vi "Write Error to File.vi"(8 "error in":errorcluster) -> ()   [LabVIEW 2021]
uses:
  <vilib>/Utility/xml.llb/Write to XML File(string).vi
panel:
  in  "message":string="An error has been occurred in the most recent NI Icon Editor session. An error report got created under the following location:\n%s"
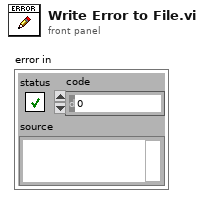
[diagram p1: front panel]
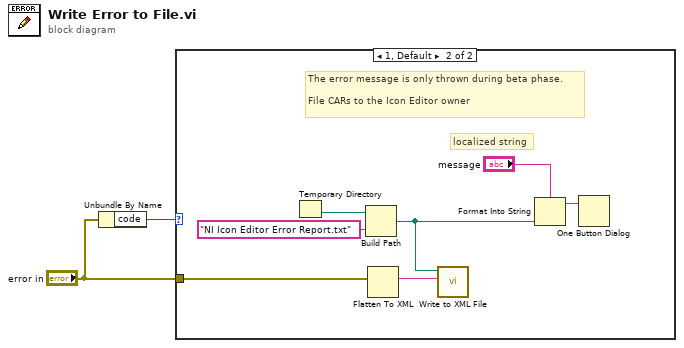
[diagram p0: block diagram]
diagram:
  n1 = Unbundle By Name("error in") -> ("code"=w2:i32)
  n2 = case shown="1, Default" w2 {
    tunnel: "error in" -> [_ w9]
    frame 0, 43 {
    }
    frame 1, Default {
      # "localized string"
      # "The error message is only thrown during beta phase.\n\nFile CARs to the Icon Editor owner"
      n3 = Temporary Directory() -> (w7:path)
      n4 = Build Path(base path=w7, name or relative path="NI Icon Editor Error Report.txt") -> (appended path=w4:path)
      n5 = Flatten To XML(6:w9) -> (2:w8:string)
      n6 = call-poly <vilib>:"Write to XML File.vi"("XML Input"=w8, "XML File Path"=w4) -> ()  [unwired: 3 in, 7 out]
      n7 = Format Into String(format string="message", w4) -> (resulting string=w3:string)  [unwired: 2 in, 1 out]
      n8 = One Button Dialog(message=w3) -> ()  [unwired: 2 out]
    }
  }
